vi "Get Name.vi"(8 "error in (no error)":errorcluster, 11 "Service in":refnum<class "Service.lvclass">) -> (0 "error out":errorcluster, 2 "Name":string, 3 "Service out":refnum<class "Service.lvclass">)   [LabVIEW 2024, in "Ramses Framework.lvlib" / "Service.lvclass"]
uses:
  Service.lvclass
  Service.lvclass/Service.ctl
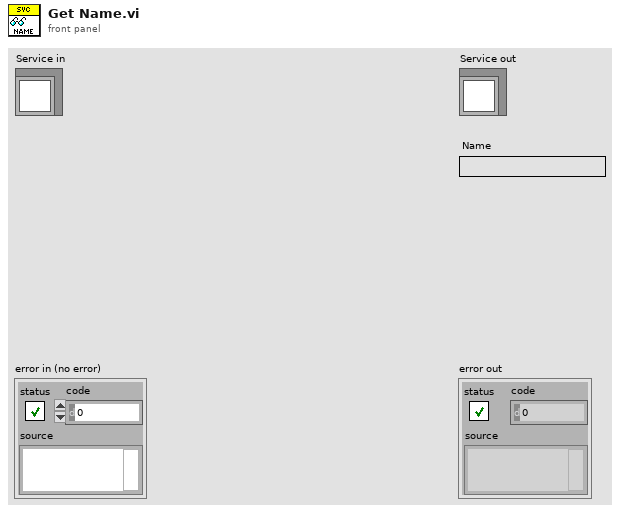
[diagram p1: front panel]
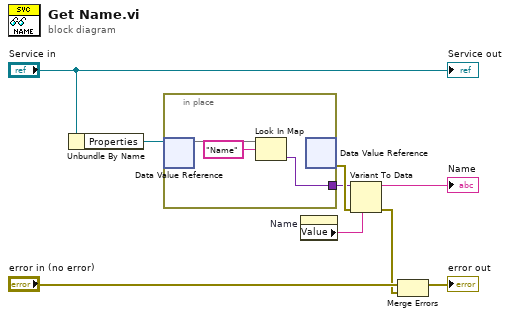
[diagram p0: block diagram]
diagram:
  n1 = Unbundle By Name("Service in") -> ("Properties"=w7:refnum<data-value>)
  n2 = in-place {
    in-place-border: [w10] -> w5
    n3 = in-place-dvr #1(w7) -> (w11:map{string, variant})  [unwired: 1 out]
    n4 = Look In Map(map=w11, key="Name" ("Key")) -> (value=w10:variant)  [unwired: 1 in, 1 out]
    n5 = in-place-dvr #1() -> (w9:errorcluster)  [unwired: 1 in, 1 out]
  }
  n6 = property on="Name" class="Str"() -> ("Value"=w4:string)  [unwired: 2 in, 2 out]
  n7 = Variant To Data(error in=w9, type=w4, Variant=w5) -> (data=→"Name":string, error out=w2:errorcluster)
  n8 = Merge Errors("error in (no error)", w2) -> (→"error out":errorcluster)
  "Service out" <- "Service in"
